vi "Register Builds Callback.vi"(7 "Owner":refnum<class>, 8 "error in (no error)":errorcluster, 10 "Callback":refnum<vi>, 11 "WebProjectWatcher in":refnum<class "WebProjectWatcher.lvclass">) -> (0 "error out":errorcluster, 3 "WebProjectWatcher out":refnum<class "WebProjectWatcher.lvclass">)   [LabVIEW 2020, in "PicoG-Processor.lvlib" / "WebProjectWatcher.lvclass"]
uses:
  WebProjectWatcher.lvclass
  Builds Callback.ctl
  WebProjectWatcher.lvclass/WebProjectWatcher.ctl
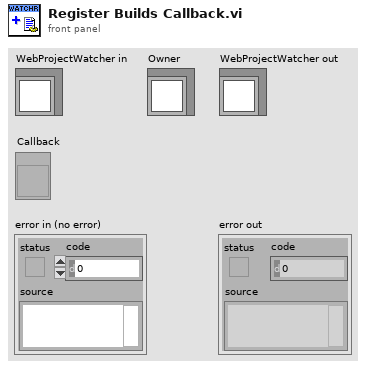
[diagram p1: front panel]
types:
  T1 = typedef "PicoG-Processor.lvlib/WebProjectWatcher.lvclass/Builds Callback.ctl" = cluster{"Callback":refnum<vi>, "Owner":refnum<class>}
  T2 = typedef "PicoG-Processor.lvlib/WebProjectWatcher.lvclass/Ref Data.ctl" = cluster{"Builds Callbacks":T1[], "Project Path":path, "Close":bool}
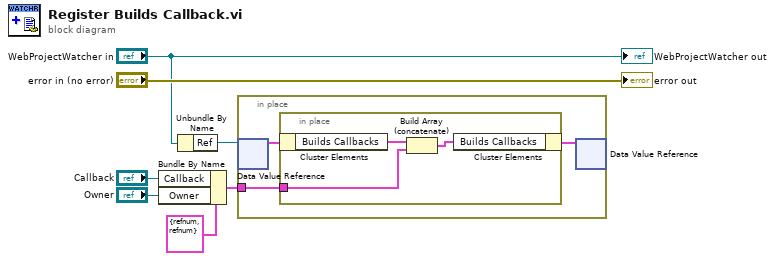
[diagram p0: block diagram]
diagram:
  n1 = Bundle By Name(cluster=T1 {"Callback"=refnum, "Owner"=refnum} ("Builds Callback"), "Callback"="Callback", "Owner"="Owner") -> (w1:T1)
  n2 = Unbundle By Name("WebProjectWatcher in") -> ("Ref"=w3:refnum<data-value>)
  n3 = in-place {
    in-place-border: w1 -> [w8]
    n4 = in-place-dvr #1(w3) -> (w10:T2)  [unwired: 1 out]
    n5 = in-place {
      in-place-border: w8 -> [w12]
      n6 = in-place-cluster #2(w10) -> ("Builds Callbacks"=w13:T1[])
      n7 = Build Array (concatenate)(w13, w12) -> (w11:T1[])
      n8 = in-place-cluster #2("Builds Callbacks"=w11) -> (w9:T2)
    }
    n9 = in-place-dvr #1(w9) -> ()  [unwired: 2 out]
  }
  "error out" <- "error in (no error)"
  "WebProjectWatcher out" <- "WebProjectWatcher in"
